vi "enumerateStaticDependencies.vi"(8 "error in (no error)":errorcluster, 11 "EmbeddedMainUI":refnum<class "EmbeddedMainUI.lvclass">) -> (0 "error out":errorcluster, 2 "Static Dependencies":refnum<class "Dependency.lvclass">[](array[class]), 3 "EmbeddedMainUI out":refnum<class "EmbeddedMainUI.lvclass">)   [LabVIEW 2016, in "EmbeddedMainUI.lvclass"]
doc: "JKI State Machine Objects (SMO) 1.3.0.56\nJKI - JKI\nCopyright (c) 2017, JKI"
uses:
  EmbeddedMainUI.lvclass
  <vilib>/JKI/JKI SMO/Dependency/Dependency.lvclass
  <vilib>/JKI/JKI SMO/SMO.UI/SMO.UI.lvclass
  <vilib>/Levylab/Embedded SMO UI/EmbeddedSMO.lvclass
  C:/Program Files (x86)/National Instruments/LabVIEW 2016/vi.lib/JKI/JKI SMO/SMO/SMO.lvclass
panel:
  # "For instructions on how to use the JKI State Machine Objects, examples and video tutorials, visit:\nhttp://jki.net/state-machine-objects/\n\nJKI State Machine Objects™\nhttp://jki.net/state-machine-objects/\nCopyright (C) 2005-2015, JKI <info@jki.net>\nALL RIGHTS RESERVED"
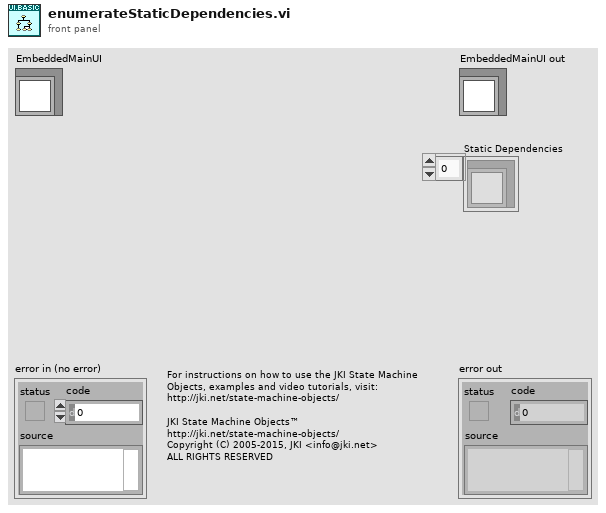
[diagram p1: front panel]
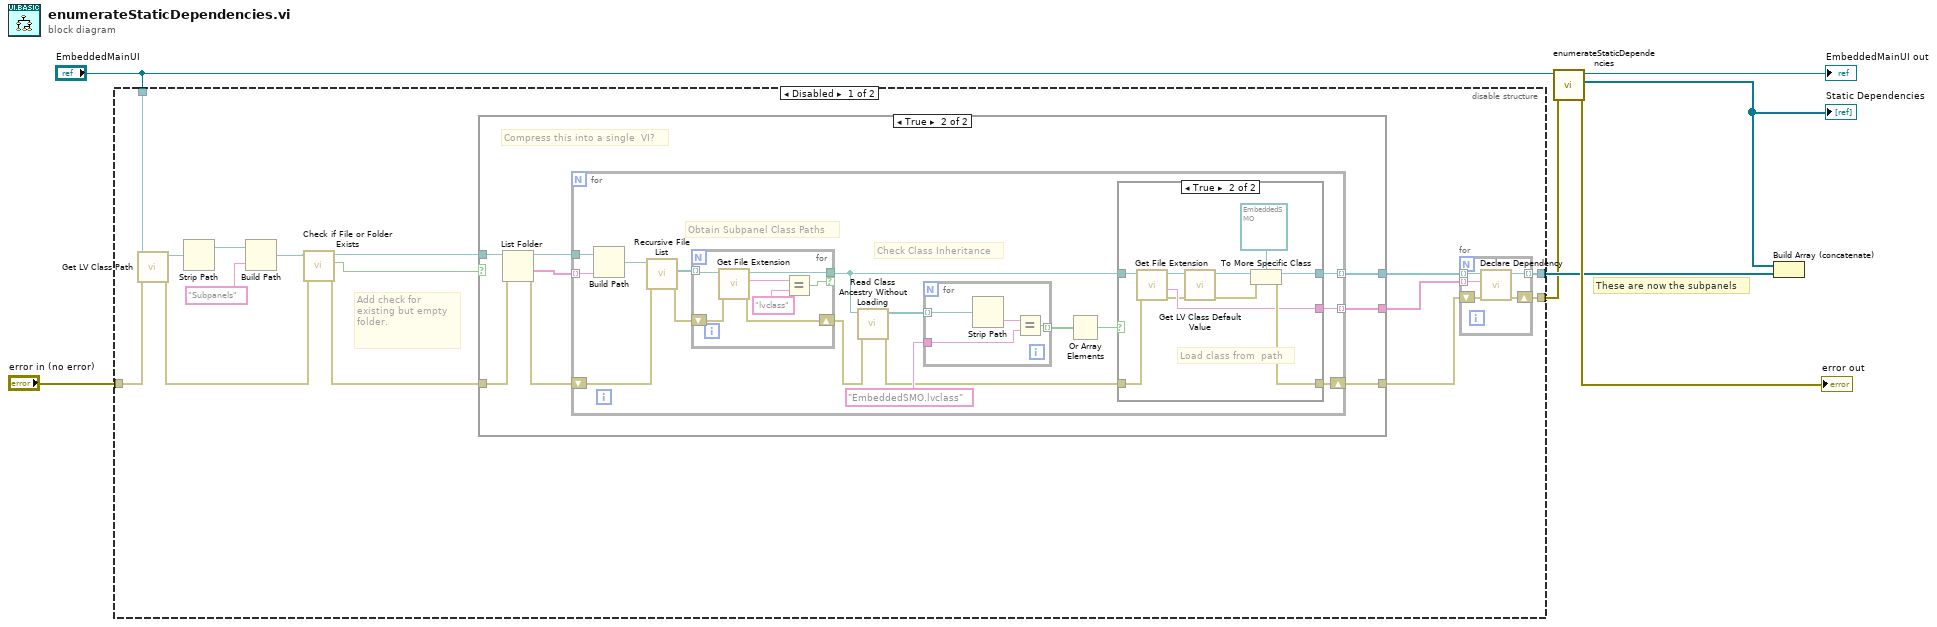
[diagram p0: block diagram]
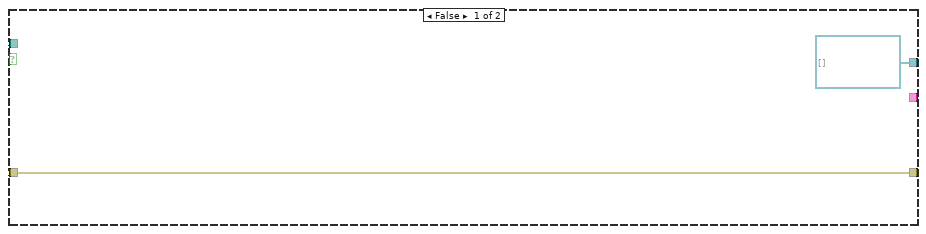
[diagram p2: hidden frame]
diagram:
  # "These are now the subpanels"
  n1 = disable-structure shown="Disabled" {
    disable-tunnel: "EmbeddedMainUI" -> [w15 _]
    disable-tunnel: "error in (no error)" -> [w12 _]
    disable-tunnel: [w10 _] -> w3
    disable-tunnel: [w8 _] -> w2
    frame Disabled {
      # "Add check for existing but empty folder."
      n2 = call <vilib>:"Get LV Class Path.vi"("error in (no error)"=w12, "object"=w15) -> ("error out"=w13:errorcluster, "class path"=w22:path)  [unwired: 8 in]
      n3 = Strip Path(path=w22) -> (stripped path=w21:path)  [unwired: 1 out]
      n4 = Build Path(base path=w21, name or relative path="Subpanels") -> (appended path=w19:path)
      n5 = call <vilib>:"Check if File or Folder Exists.vi"("error in (no error)"=w13, "path"=w19) -> ("error out"=w17:errorcluster, "file or folder exists?"=w16:bool, "dup path"=w18:path)  [unwired: 7 in]
      n6 = case shown="True" w16 {
        tunnel: w18 -> [w30 w38]
        tunnel: w17 -> [w29 w33]
        tunnel: [w29 w32] -> w9
        tunnel: [refnum<class "EmbeddedSMO.lvclass">[] [] w34] -> w14
        tunnel: [_ w31] -> w11
        frame False {
          n7 = Create Folder(path (use dialog)=w30, error in=w29) -> ()  [unwired: 1 in, 3 out]
        }
        frame True {
          # "Compress this into a single  VI?"
          n8 = List Folder(path=w38, error in=w33) -> (path out=w37:path, folder names=w36:string[], error out=w35:errorcluster)  [unwired: 2 in, 1 out]
          n9 = for {
            tunnel: w37 -> [w54]
            tunnel: w36 -> [w53] mode=indexing
            tunnel: [w49] -> w34 mode=indexing
            shift-right: [w41] -> w32
            shift-left: w35 -> [w45]
            tunnel: [w39] -> w31 mode=indexing
            # "Check Class Inheritance"
            # "Obtain Subpanel Class Paths"
            n10 = Build Path(base path=w54, name or relative path=w53) -> (appended path=w52:path)
            n11 = call <vilib>:"Recursive File List.vi"("error in (no error)"=w45, "Folder Path"=w52) -> ("error out"=w44:errorcluster, "All Files in Dir"=w51:path[])  [unwired: 5 in, 3 out]
            n12 = for {
              tunnel: w51 -> [w74] mode=indexing
              tunnel: [w73] -> w50 if=w72
              shift-right: [w70] -> w43
              shift-left: w44 -> [w71]
              n13 = call <vilib>:"Get File Extension.vi"("error in (no error)"=w71, "file"=w74) -> ("error out"=w70:errorcluster, "lowercase file extension"=w76:string, "dup file"=w73:path)  [unwired: 5 in, 2 out]
              n14 = Equal?(x=w76, y="lvclass") -> (x = y?=w72:bool)
            }
            n15 = call <vilib>:"Read Class Ancestry Without Loading.vi"("error in (no error)"=w43, "LabVIEW Class Path"=w50) -> ("error out"=w42:errorcluster, "Class Ancestry"=w48:path[])  [unwired: 8 in]
            n16 = for {
              tunnel: w48 -> [w69] mode=indexing
              tunnel: [w67] -> w47 mode=indexing
              tunnel: "EmbeddedSMO.lvclass" -> [w66]
              n17 = Strip Path(path=w69) -> (name=w68:string)  [unwired: 1 out]
              n18 = Equal?(x=w68, y=w66) -> (x = y?=w67:bool)
            }
            n19 = Or Array Elements(Boolean array=w47) -> (logical OR=w40:bool)
            n20 = case shown="True" w40 {
              tunnel: w50 -> [_ w60]
              tunnel: [_ w65] -> w49
              tunnel: w42 -> [w55 w57]
              tunnel: [w55 w61] -> w41
              tunnel: [_ w58] -> w39
              frame False {
              }
              frame True {
                # "Load class from  path"
                n21 = call <vilib>:"Get File Extension.vi"("error in (no error)"=w57, "file"=w60) -> ("error out"=w56:errorcluster, "filename without extension"=w58:string, "dup file"=w59:path)  [unwired: 5 in, 2 out]
                n22 = call <vilib>:"Get LV Class Default Value.vi"("error in (no error)"=w56, "class path"=w59) -> ("error out"=w62:errorcluster, "object"=w64:refnum<class>)  [unwired: 8 in]
                n23 = To More Specific Class(target class=refnum<class "EmbeddedSMO.lvclass"> refnum ("EmbeddedSMO"), reference=w64, error in=w62) -> (specific class reference=w65:refnum<class "EmbeddedSMO.lvclass">, error out=w61:errorcluster)
              }
            }
          }
        }
      }
      n24 = for {
        tunnel: w14 -> [w27] mode=indexing
        tunnel: [w26] -> w10 mode=indexing
        tunnel: w11 -> [w25] mode=indexing
        shift-right: [w23] -> w8
        shift-left: w9 -> [w24]
        n25 = call <vilib>:"Declare Dependency.vi"("error in (no error)"=w24, "Name"=w25, "Type"=w27) -> ("error out"=w23:errorcluster, "Dependency out"=w26:refnum<class "Dependency.lvclass">)  [unwired: 7 in]
      }
    }
    frame Enabled {
    }
  }
  n26 = call-parent "enumerateStaticDependencies.vi"("error in (no error)"=w2, "SMO"="EmbeddedMainUI") -> ("error out"=→"error out":errorcluster, "Static Dependencies"=w1:refnum<class "Dependency.lvclass">[], "SMO out"=→"EmbeddedMainUI out":refnum<class "EmbeddedMainUI.lvclass">)  [unwired: 7 in]
  "Static Dependencies" <- w1
  n27 = Build Array (concatenate)(w1, w3) -> ()  [unwired: 1 out]
